vi "Tanget of Waypoint Segment.vi"(9 "point c":cluster{"x":sgl, "y":sgl}, 10 "point b":cluster{"x":sgl, "y":sgl}, 11 "point a":cluster{"x":sgl, "y":sgl}) -> (3 "T_i":cluster{sgl, sgl})   [LabVIEW 2025]
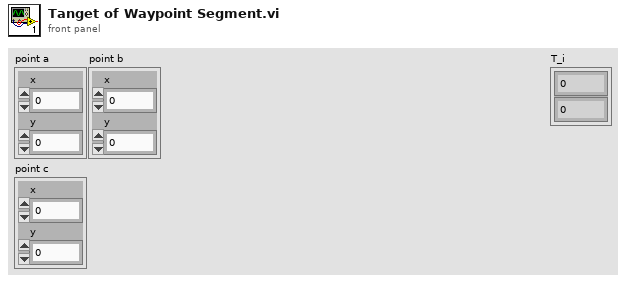
[diagram p1: front panel]
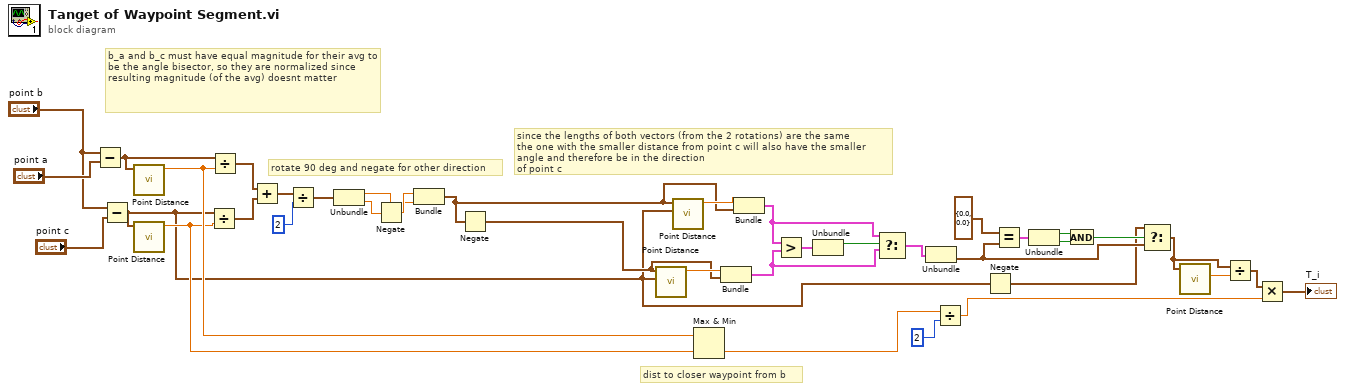
[diagram p0: block diagram]
diagram:
  # "b_a and b_c must have equal magnitude for their avg to be the angle bisector, so they are normalized since resulting magnitude (of the avg) doesnt matter"
  # "dist to closer waypoint from b"
  # "since the lengths of both vectors (from the 2 rotations) are the same\nthe one with the smaller distance from point c will also have the smaller angle and therefore be in the direction\nof point c"
  # "rotate 90 deg and negate for other direction"
  n1 = Subtract(x="point b", y="point a") -> (x-y=w37:cluster{"x":sgl, "y":sgl})
  n2 = Subtract(x="point b", y="point c") -> (x-y=w7:cluster{"x":sgl, "y":sgl})
  n3 = call "Point Distance.vi"("point a"=w37) -> ("dist"=w23:sgl)  [unwired: 10 in]
  n4 = call "Point Distance.vi"("point a"=w7) -> ("dist"=w22:sgl)  [unwired: 10 in]
  n5 = Divide(x=w7, y=w22) -> (x/y=w35:cluster{"x":sgl, "y":sgl})
  n6 = Divide(x=w37, y=w23) -> (x/y=w36:cluster{"x":sgl, "y":sgl})
  n7 = Add(x=w36, y=w35) -> (x+y=w34:cluster{"x":sgl, "y":sgl})
  n8 = Divide(x=w34, y=u16 2) -> (x/y=w32:cluster{"x":sgl, "y":sgl})
  n9 = Unbundle(w32) -> ("x"=w29:sgl, "y"=w31:sgl)
  n10 = Negate(x=w31) -> (-x=w30:sgl)
  n11 = Bundle(w30, "x"=w29) -> (w18:cluster{sgl, "x":sgl})  [unwired: 1 in]
  n12 = Negate(x=w18) -> (-x=w17:cluster{sgl, "x":sgl})
  n13 = call "Point Distance.vi"("point b"=w7, "point a"=w17) -> ("dist"=w26:sgl)  [unwired: 9 in]
  n14 = call "Point Distance.vi"("point b"=w7, "point a"=w18) -> ("dist"=w27:sgl)  [unwired: 9 in]
  n15 = Max & Min(x=w23, y=w22) -> (min(x,y)=w21:sgl)  [unwired: 1 out]
  n16 = Bundle("dist"=w26, w17) -> (w2:cluster{"dist":sgl, cluster{sgl, "x":sgl}})  [unwired: 1 in]
  n17 = Bundle("dist"=w27, w18) -> (w3:cluster{"dist":sgl, cluster{sgl, "x":sgl}})  [unwired: 1 in]
  n18 = Greater?(x=w3, y=w2) -> (0:w5:cluster{"dist":bool, cluster{bool, "x":bool}})
  n19 = Unbundle(w5) -> ("dist"=w4:bool)  [unwired: 1 out]
  n20 = Select(t=w3, s=w4, f=w2) -> (s? t:f=w1:cluster{"dist":sgl, cluster{sgl, "x":sgl}})
  n21 = Unbundle(w1) -> (w10:cluster{sgl, "x":sgl})  [unwired: 1 out]
  n22 = Divide(x=w21, y=u16 2) -> (x/y=w25:sgl)
  n23 = Negate(x=w7) -> (-x=w6:cluster{"x":sgl, "y":sgl})
  n24 = Equal?(x=cluster{dbl, "x":dbl} {0.0, "x"=0.0}, y=w10) -> (x = y?=w13:cluster{bool, "x":bool})
  n25 = Unbundle(w13) -> (w12:bool, "x"=w11:bool)
  n26 = And(x=w12, y=w11) -> (x .and. y?=w9:bool)
  n27 = Select(t=w6, s=w9, f=w10) -> (s? t:f=w8:cluster{"x":sgl, "x":sgl})
  n28 = call "Point Distance.vi"("point a"=w8) -> ("dist"=w20:sgl)  [unwired: 10 in]
  n29 = Divide(x=w8, y=w20) -> (x/y=w19:cluster{"x":sgl, "x":sgl})
  n30 = Multiply(x=w19, y=w25) -> (x*y=→"T_i":cluster{"x":sgl, "x":sgl})
